vi "Pre-Command.vi"(8 "error in (no error)":errorcluster, 10 "command in":T2, 11 "Thread in":refnum<class "Thread.lvclass">) -> (0 "error out":errorcluster, 2 "command out":T2, 3 "Thread out":refnum<class "Thread.lvclass">, 5 "state":T1)   [LabVIEW 2017, in "DSF Core.lvlib" / "Thread.lvclass"]
uses:
  Thread.lvclass
  Thread Command.ctl
  Thread State.ctl
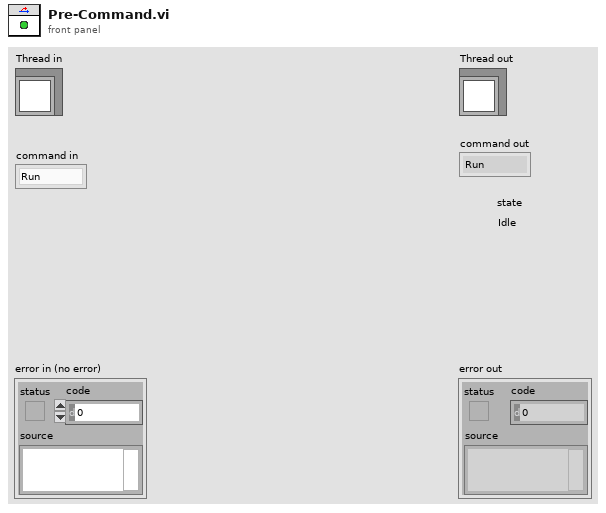
[diagram p1: front panel]
types:
  T1 = typedef "DSF Core.lvlib/Thread.lvclass/Thread State.ctl" = enum8{"Idle", "Running", "Error", "Shut Down"}
  T2 = typedef "DSF Core.lvlib/Thread.lvclass/Thread Command.ctl" = enum8{"Run", "Shutdown"}
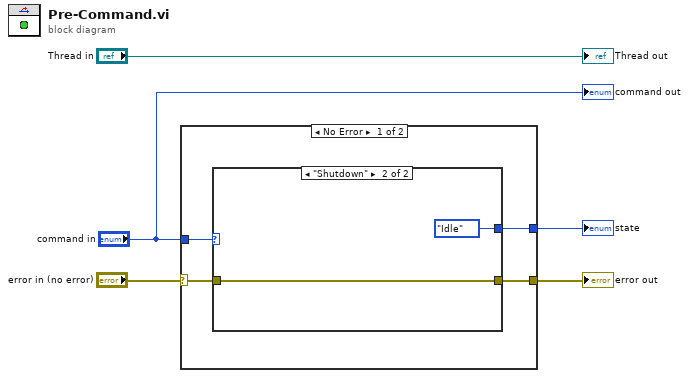
[diagram p0: block diagram]
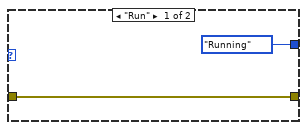
[diagram p2: hidden frame]
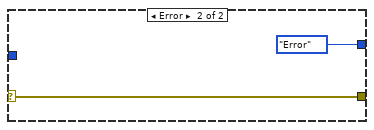
[diagram p3: hidden frame]
diagram:
  n1 = case shown="No Error" "error in (no error)" {
    selector: "error in (no error)" -> [w8 w15]
    tunnel: [w7 w15] -> w4
    tunnel: [w6 Thread_State."Error" ("State")] -> w1
    tunnel: "command in" -> [w9 _]
    frame No Error {
      n2 = case shown="\"Shutdown\"" w9 {
        tunnel: w8 -> [w11 w12]
        tunnel: [w11 w12] -> w7
        tunnel: [Thread_State."Running" ("State") Thread_State."Idle" ("State")] -> w6
        frame "Run" {
        }
        frame "Shutdown" {
        }
      }
    }
    frame Error {
    }
  }
  "error out" <- w4
  "state" <- w1
  "Thread out" <- "Thread in"
  "command out" <- "command in"
